vi "BRig_dataBlock_c_T2R_L.vi"() -> (2 "output_c_T2R_L":i32)   [LabVIEW 2014]
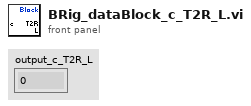
[diagram p1: front panel]
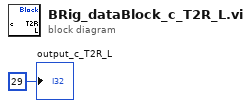
[diagram p0: block diagram]
diagram:
  "output_c_T2R_L" <- 29 ("output_iBlock")
